vi "Refresh Tree.vi"(8 "error in (no error)":errorcluster, 10 "Include Dependencies?":bool, 11 "Message Maker in":refnum<class "Message Maker.lvclass">) -> (0 "error out":errorcluster, 1 "Messages out of date?":bool, 3 "Message Maker out":refnum<class "Message Maker.lvclass">)   [LabVIEW 2023, in "Message Maker.lvclass"]
doc: "Refreshes the status of the tree. This will find all actors and their callable methods\n\nAuthor: Derek Trepanier\nCopyright: MGI 2015"
uses:
  Message Maker.lvclass
  Details Map.ctl
  Message Maker.lvclass/Message Maker.ctl
  Message Status.ctl
  Is an Actor-Interface.vi
  Get Message Status.vi
panel:
  in  "Details Map":T1
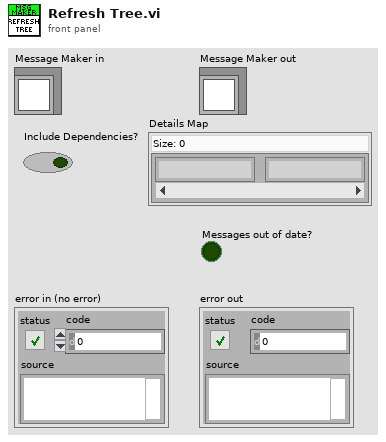
[diagram p1: front panel]
types:
  T1 = typedef "Message Maker.lvclass/Details Map.ctl" = map{string, string}
  T2 = typedef "Message Maker.lvclass/Message Status.ctl" = enum16{"Message Not Created", "Message Out of Date", "Message OK", "Never update"}
  T3 = enum8{"Enabled", "Disabled", "Disabled and Grayed Out"}
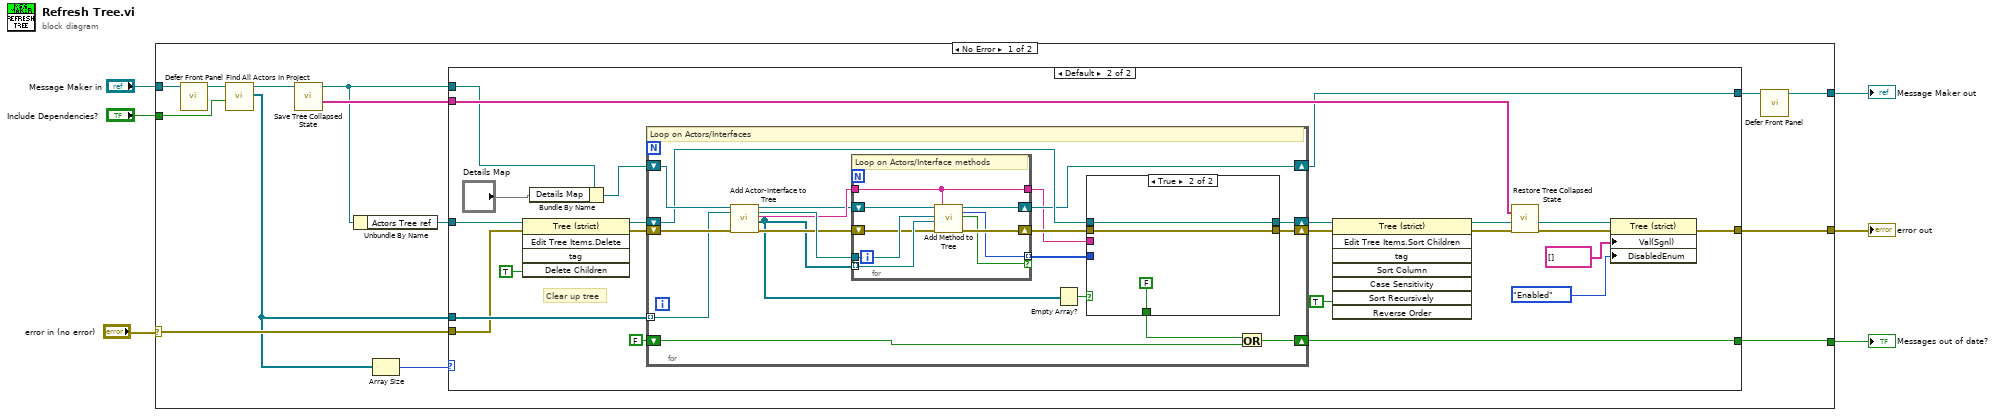
[diagram p0: block diagram]
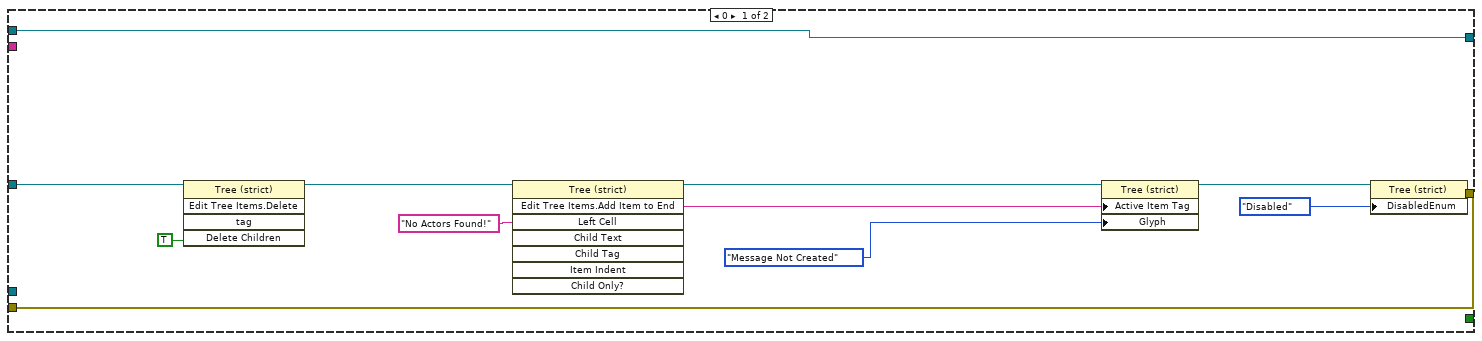
[diagram p2: hidden frame]
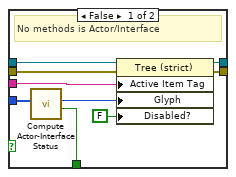
[diagram p3: hidden frame]
diagram:
  n1 = case shown="No Error" "error in (no error)" {
    selector: "error in (no error)" -> [w18 w95]
    tunnel: [w14 w95] -> w6
    tunnel: [w19 w96] -> w5
    tunnel: "Message Maker in" -> [w17 w96]
    tunnel: "Include Dependencies?" -> [w11 _]
    tunnel: [w15 _] -> w1
    frame No Error {
      n2 = call "Defer Front Panel.vi"("Message Maker in"=w17) -> ("Message Maker out"=w13:refnum<class "Message Maker.lvclass">)  [unwired: 9 in, 1 out]
      n3 = call "Find All Actors In Project.vi"("Include Dependencies?"=w11, "Message Maker in"=w13) -> ("Actor Classes"=w12:refnum<vi>[], "Message Maker out"=w10:refnum<class "Message Maker.lvclass">)  [unwired: 7 in, 1 out]
      n4 = call "Save Tree Collapsed State.vi"("Message Maker in"=w10) -> ("Array"=w16:string[], "Message Maker out"=w8:refnum<class "Message Maker.lvclass">)  [unwired: 9 in]
      n5 = Unbundle By Name(w8) -> ("Actors Tree ref"=w7:refnum<vi>)
      n6 = Array Size(array=w12) -> (size(s)=w20:i32)
      n7 = case shown="Default" w20 {
        tunnel: w12 -> [_ w54]
        tunnel: w7 -> [w30 w53]
        tunnel: w18 -> [w31 w52]
        tunnel: [w31 w45] -> w14
        tunnel: w16 -> [_ w39]
        tunnel: [_ w37] -> w15
        tunnel: w8 -> [w21 w35]
        tunnel: [w21 w33] -> w9
        frame 0 {
          n8 = invoke class="Tree (strict)" method="Edit Tree Items.Delete"(reference=w30, "Delete Children"=TRUE ("Delete Children?")) -> (reference out=w28:refnum<vi>)  [unwired: 3 in, 4 out]
          n9 = invoke class="Tree (strict)" method="Edit Tree Items.Add Item to End"(reference=w28, "Left Cell"="No Actors Found!" ("Left Cell String")) -> (reference out=w25:refnum<vi>, "Edit Tree Items:Add Item to End"=w23:string)  [unwired: 6 in, 6 out]
          n10 = property on="Property Node" class="Tree (strict)"(reference=w25, "Active Item Tag"=w23, "Glyph"=Message_Status."Message Not Created" ("Enum")) -> (reference out=w24:refnum<vi>)  [unwired: 1 in, 1 out]
          n11 = property class="Tree (strict)"(reference=w24, "DisabledEnum"=T3."Disabled" ("Disabled")) -> ()  [unwired: 1 in, 2 out]
        }
        frame Default {
          # "Clear up tree"
          n12 = invoke class="Tree (strict)" method="Edit Tree Items.Delete"(reference=w53, error in=w52, "Delete Children"=TRUE ("Delete Children?")) -> (reference out=w49:refnum<vi>, error out=w51:errorcluster)  [unwired: 2 in, 3 out]
          n13 = Bundle By Name(cluster=w35, "Details Map"="Details Map") -> (w34:refnum<class "Message Maker.lvclass">)
          n14 = for {
            tunnel: w54 -> [w72] mode=indexing
            shift-right: [w70] -> w48
            shift-left: w49 -> [w59]
            shift-right: [w69] -> w47
            shift-left: w51 -> [w73]
            shift-right: [w65] -> w37
            shift-left: FALSE -> [w64]
            shift-right: [w58] -> w33
            shift-left: w34 -> [w61]
            # "Loop on Actors/Interfaces"
            n15 = call "Add Actor-Interface to Tree.vi"("Message Maker in"=w61, "Actor/Interface Refnum in"=w72, "error in (no error)"=w73) -> ("Message Maker out"=w60:refnum<class "Message Maker.lvclass">, "Actor/Interface Refnum out"=w71:refnum<vi>, "Edit Tree Items:Add Item to End"=w62:string, "All Method Refnums"=w56:refnum<vi>[], "error out"=w63:errorcluster)  [unwired: 12 in]
            n16 = for {
              shift-right: [w92] -> w58
              shift-left: w60 -> [w94]
              tunnel: w56 -> [w93] mode=indexing
              tunnel: w62 -> [w87]
              shift-right: [w91] -> w68
              shift-left: w63 -> [w88]
              tunnel: w71 -> [w90]
              tunnel: [w89] -> w67 mode=indexing if=w86
              tunnel: [w87] -> w57
              # "Loop on Actors/Interface methods"
              n17 = call "Add Method to Tree.vi"("Message Maker in"=w94, "Actor/Interface Refnum"=w90, "Method VI Refnum"=w93, "error in (no error)"=w88, "Actor/Interface Tag"=w87) -> ("Message Maker out"=w92:refnum<class "Message Maker.lvclass">, "Message Status"=w89:T2, "Is Public Method"=w86:bool, "error out"=w91:errorcluster)  [unwired: 11 in]
            }
            n18 = Empty Array?(array=w56) -> (empty?=w55:bool)
            n19 = case shown="True" w55 {
              tunnel: [w82 w84] -> w70
              tunnel: [w81 w83] -> w69
              tunnel: w68 -> [w80 w83]
              tunnel: w67 -> [w78 _]
              tunnel: [w77 FALSE ("Any Message Out of Date?")] -> w66
              tunnel: w59 -> [w75 w84]
              tunnel: w57 -> [w74 _]
              frame False {
                # "No methods is Actor/Interface"
                n20 = call "Compute Actor-Interface Status.vi"("Array"=w78) -> ("Any Message Out of Date?"=w77:bool, "Actor/Interface Status"=w79:T2)  [unwired: 9 in]
                n21 = property on="Property Node" class="Tree (strict)"(reference=w75, error in=w80, "Active Item Tag"=w74, "Glyph"=w79, "Disabled?"=FALSE ("Active Item:Disabled?")) -> (reference out=w82:refnum<vi>, error out=w81:errorcluster)
              }
              frame True {
              }
            }
            n22 = Or(x=w66, y=w64) -> (x .or. y?=w65:bool)
          }
          n23 = invoke class="Tree (strict)" method="Edit Tree Items.Sort Children"(reference=w48, error in=w47, "Sort Recursively"=TRUE ("Sort Recursively?")) -> (reference out=w43:refnum<vi>, error out=w42:errorcluster)  [unwired: 5 in, 6 out]
          n24 = call "Restore Tree Collapsed State.vi"("TreeControl in"=w43, "Array"=w39, "error in (no error)"=w42) -> ("TreeControl out"=w41:refnum<vi>, "error out"=w40:errorcluster)  [unwired: 15 in]
          n25 = property class="Tree (strict)"(reference=w41, error in=w40, "Val(Sgnl)"=string[] [] ("Value (Signaling)"), "DisabledEnum"=T3."Enabled" ("Disabled")) -> (error out=w45:errorcluster)  [unwired: 1 out]
        }
      }
      n26 = call "Defer Front Panel.vi"("Message Maker in"=w9) -> ("Message Maker out"=w19:refnum<class "Message Maker.lvclass">)  [unwired: 9 in, 1 out]
    }
    frame Error {
    }
  }
  "error out" <- w6
  "Message Maker out" <- w5
  "Messages out of date?" <- w1
